vi "Verifiy Reset Blink Pattern.vi"(8 "Error in":errorcluster caption="Error in (no error)") -> (0 "Error out":errorcluster, 3 "Pass":bool)   [LabVIEW 2015, in "Rocom Reset.lvclass"]
uses:
  Rocom Reset/Rocom Reset.lvclass
panel:
  out "LED":bool=TRUE
  in  "Fail":bool
  in  "Pass":bool=TRUE
  # "Reset Verification"
  # "Verify the RESET blink pattern"
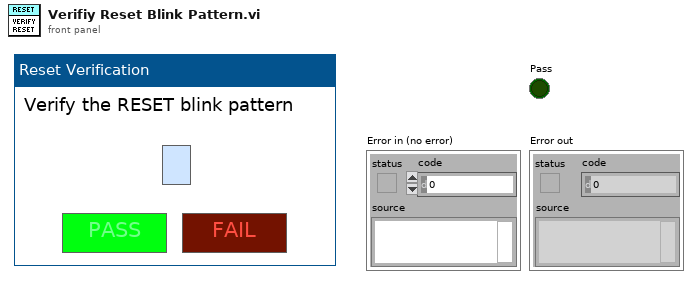
[diagram p1: front panel]
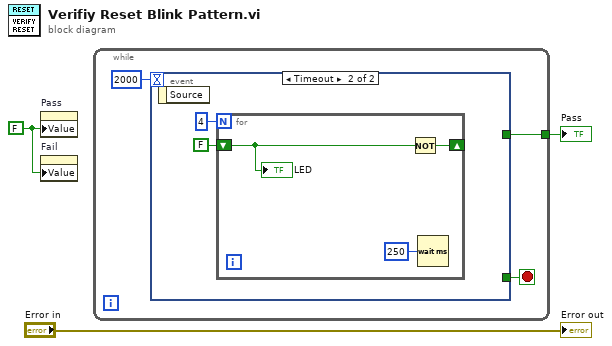
[diagram p0: block diagram]
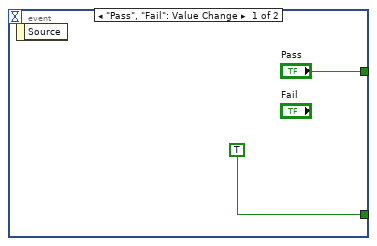
[diagram p2: hidden frame]
diagram:
  w1 = FALSE ("LED State")
  n1 = property on="Pass" class="Bool (strict)"("Value"=w1) -> ()  [unwired: 2 in, 2 out]
  n2 = property on="Fail" class="Bool (strict)"("Value"=w1) -> ()  [unwired: 2 in, 2 out]
  n3 = while {
    tunnel: [w6] -> w3
    stop <- w5 stop-if-true
    n4 = event shown="[1] Timeout" {
      selector: _ -> [_ _]
      dyn-events: _ -> [_ _]
      timeout: 2000 -> [_ _]
      tunnel: ["Pass" _] -> w6
      tunnel: [TRUE _] -> w5
      event "Pass", "Fail": Value Change {
        n5 = event-data() -> ()  [unwired: 1 in, 1 out]
      }
      event Timeout {
        n6 = event-data() -> ()  [unwired: 1 in, 1 out]
        n7 = for {
          N: 4 -> [_]
          shift-right: [w13] -> _
          shift-left: FALSE ("LED State") -> [w11]
          n8 = Not(x=w11) -> (.not. x?=w13:bool)
          n9 = Wait (ms)(milliseconds to wait=u32 250) -> ()  [unwired: 1 out]
          "LED" <- w11
        }
      }
    }
  }
  "Pass" <- w3
  "Error out" <- "Error in"
